vi "GetProperties.vi"(8 "error in":errorcluster, 11 "Text in":refnum<class "Text.lvclass">) -> (0 "error out":errorcluster, 3 "Text out":refnum<class "Text.lvclass">)   [LabVIEW 2014, in "Text.lvclass"]
uses:
  Text.lvclass
  Text.lvclass/Text.ctl
  Decoration/Decoration.lvclass
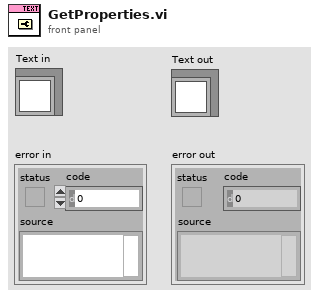
[diagram p1: front panel]
types:
  T1 = typedef "LVBoundsTypeDef.ctl" = cluster{"Width":u32, "Height":u32}
  T2 = typedef "LVFontTypeDef.ctl" = cluster{"Font Name":string, "Size":u16, "Bold":bool, "Italic":bool, "Underline":bool, "Strikeout":bool, "Color":u32}
  T3 = typedef "LVTextColorsTypeDef.ctl" = cluster{"Text Color":u32, "Background Color":u32}
  T4 = enum16{"None", "Stacked", "Clockwise", "Counterclockwise"}
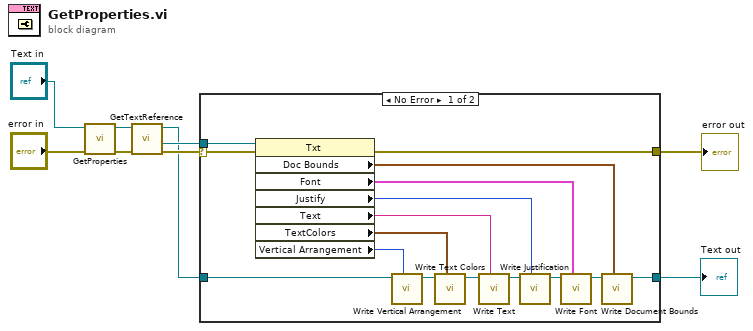
[diagram p0: block diagram]
diagram:
  n1 = call-parent "GetProperties.vi"("error in"="error in", "Decoration in"="Text in") -> ("error out"=w6:errorcluster, "Decoration out"=w7:refnum<class "Text.lvclass">)  [unwired: 8 in]
  n2 = call "GetTextReference.vi"("error in"=w6, "Decoration in"=w7) -> ("error out"=w5:errorcluster, "Text reference"=w4:refnum<vi>, "Decoration out"=w3:refnum<class "Text.lvclass">)  [unwired: 7 in]
  n3 = case shown="No Error" w5 {
    selector: w5 -> [w24 w27]
    tunnel: [w19 w27] -> w1
    tunnel: [w13 w26] -> w2
    tunnel: w3 -> [w17 w26]
    tunnel: w4 -> [w25 _]
    frame No Error {
      n4 = property class="Txt"(reference=w25, error in=w24) -> (error out=w19:errorcluster, "Doc Bounds"=w23:T1, "Font"=w10:T2, "Justify"=w22:enum16{"Left", "Center", "Right"}, "Text"=w21:string, "TextColors"=w20:T3, "Vertical Arrangement"=w18:T4)  [unwired: 1 out]
      n5 = call "Write Vertical Arrangement.vi"("Vertical Arrangement"=w18, "Text in"=w17) -> ("Text out"=w16:refnum<class "Text.lvclass">)  [unwired: 7 in]
      n6 = call "Write Text Colors.vi"("Text Colors"=w20, "Text in"=w16) -> ("Text out"=w15:refnum<class "Text.lvclass">)  [unwired: 7 in]
      n7 = call "Write Text.vi"("Text"=w21, "Text in"=w15) -> ("Text out"=w14:refnum<class "Text.lvclass">)  [unwired: 7 in]
      n8 = call "Write Justification.vi"("Justification"=w22, "Text in"=w14) -> ("Text out"=w12:refnum<class "Text.lvclass">)  [unwired: 7 in]
      n9 = call "Write Font.vi"("Font"=w10, "Text in"=w12) -> ("Text out"=w11:refnum<class "Text.lvclass">)  [unwired: 7 in]
      n10 = call "Write Document Bounds.vi"("Document Bounds"=w23, "Text in"=w11) -> ("Text out"=w13:refnum<class "Text.lvclass">)  [unwired: 7 in]
    }
    frame Error {
    }
  }
  "error out" <- w1
  "Text out" <- w2
